vi "Execute.vi"(8 "error in (no error)":errorcluster, 10 "System in":refnum<class "System.lvclass">, 11 "Command in":refnum<class "Command.lvclass">) -> (0 "error out":errorcluster, 3 "Command out":refnum<class "Command.lvclass">)   [LabVIEW 2013, in "Command.lvclass"]
uses:
  Command.lvclass
  Systems/System/System.lvclass
  Command.lvclass/Command.ctl
  States/State/State.lvclass
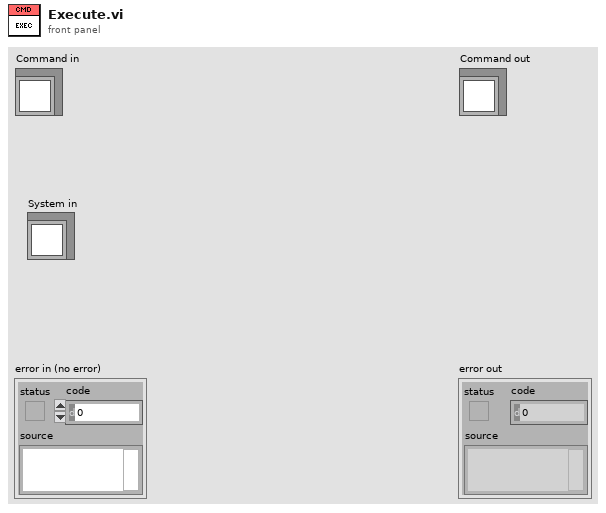
[diagram p1: front panel]
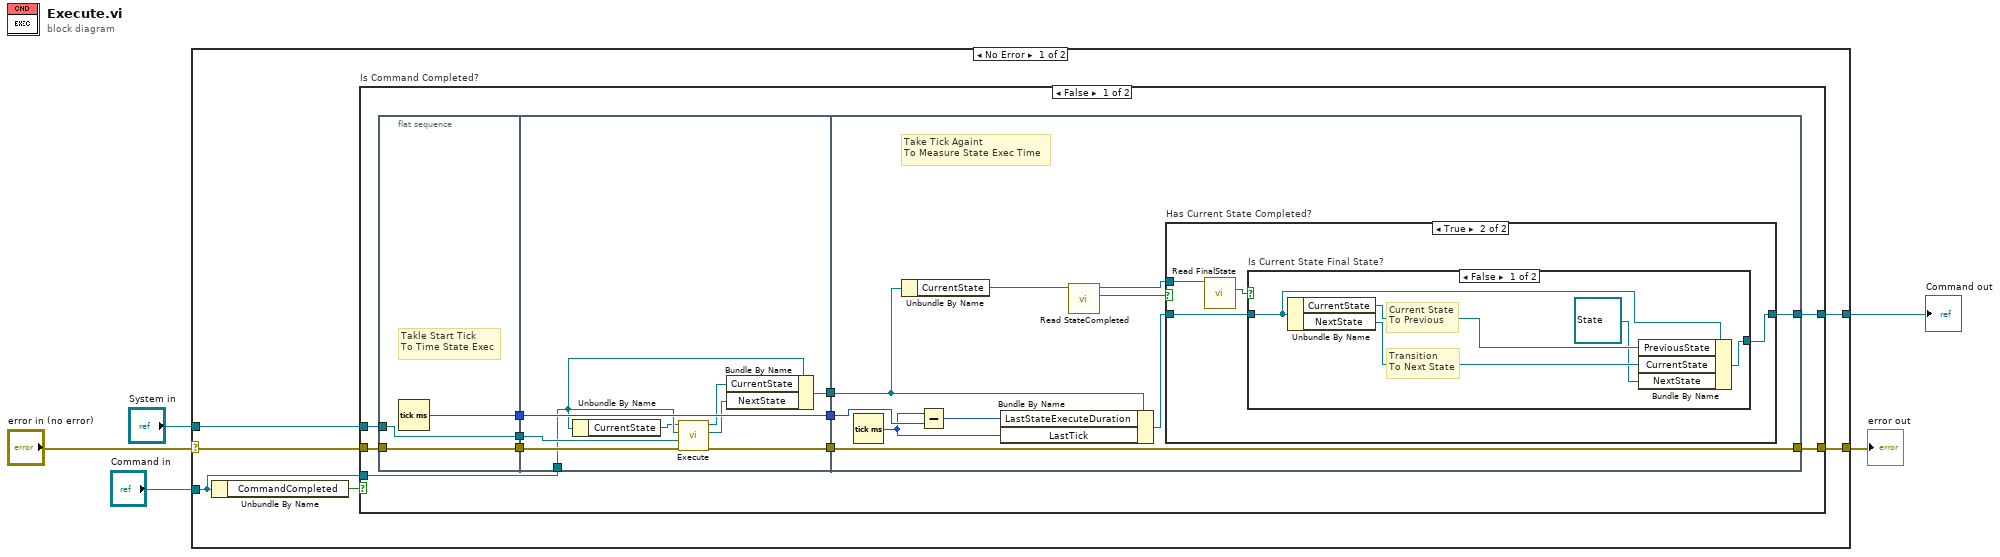
[diagram p0: block diagram]
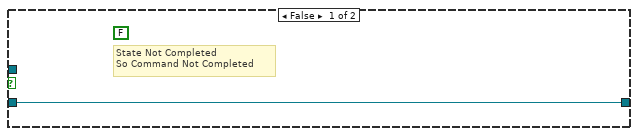
[diagram p2: hidden frame]
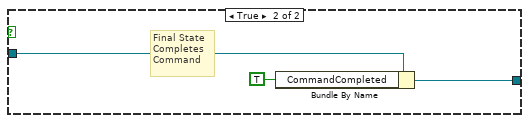
[diagram p3: hidden frame]
diagram:
  n1 = case shown="No Error" "error in (no error)" {
    selector: "error in (no error)" -> [w8 w61]
    tunnel: [w7 w61] -> w4
    tunnel: [w9 w60] -> w2
    tunnel: "Command in" -> [w10 w60]
    tunnel: "System in" -> [w6 _]
    frame No Error {
      n2 = Unbundle By Name(w10) -> ("CommandCompleted"=w11:bool)
      n3 = case "Is Command Completed?" shown="False" w11 {
        tunnel: w10 -> [w13 w58]
        tunnel: [w12 w58] -> w9
        tunnel: w8 -> [w22 w59]
        tunnel: [w21 w59] -> w7
        tunnel: w6 -> [w20 _]
        frame False {
          n4 = flat-sequence {
            tunnel: w20 -> [w24]
            tunnel: w22 -> [w25]
            tunnel: [w25] -> w18
            tunnel: [w24] -> w17
            tunnel: [w23] -> w14
            tunnel: [w33] -> w19
            tunnel: w18 -> [w34]
            tunnel: w17 -> [w32]
            tunnel: [w28] -> w16
            tunnel: [w31] -> w15
            tunnel: w14 -> [w31]
            tunnel: w13 -> [w30]
            tunnel: [w44] -> w21
            tunnel: w19 -> [w44]
            tunnel: w16 -> [w36]
            tunnel: [w38] -> w12
            tunnel: w15 -> [w43]
            frame #0 {
              # "Takle Start Tick\nTo Time State Exec"
              n5 = Tick Count (ms)() -> (millisecond timer value=w23:u32)
            }
            frame #1 {
              n6 = Unbundle By Name(w30) -> ("CurrentState"=w29:refnum<class "State.lvclass">)
              n7 = call-dynamic "Execute.vi"("error in (no error)"=w34, "System in"=w32, "Command in"=w30, "State in"=w29) -> ("error out"=w33:errorcluster, "Next State"=w27:refnum<class "State.lvclass">, "State out"=w26:refnum<class "State.lvclass">)  [unwired: 5 in]
              n8 = Bundle By Name(cluster=w30, "CurrentState"=w26, "NextState"=w27) -> (w28:refnum<class "Command.lvclass">)
            }
            frame #2 {
              # "Take Tick Againt\nTo Measure State Exec Time"
              n9 = Tick Count (ms)() -> (millisecond timer value=w37:u32)
              n10 = Unbundle By Name(w36) -> ("CurrentState"=w35:refnum<class "State.lvclass">)
              n11 = Subtract(x=w37, y=w43) -> (x-y=w42:u32)
              n12 = Bundle By Name(cluster=w36, "LastStateExecuteDuration"=w42, "LastTick"=w37) -> (w39:refnum<class "Command.lvclass">)
              n13 = call-dynamic "Read StateCompleted.vi"("State in"=w35) -> ("StateCompleted"=w41:bool, "State out"=w40:refnum<class "State.lvclass">)  [unwired: 8 in, 1 out]
              n14 = case "Has Current State Completed?" shown="True" w41 {
                tunnel: w39 -> [w45 w47]
                tunnel: w40 -> [_ w49]
                tunnel: [w45 w46] -> w38
                frame False {
                  (unwired) FALSE
                  # "State Not Completed\nSo Command Not Completed"
                }
                frame True {
                  n15 = call-dynamic "Read FinalState.vi"("State in"=w49) -> ("FinalState"=w48:bool)  [unwired: 8 in, 2 out]
                  n16 = case "Is Current State Final State?" shown="False" w48 {
                    tunnel: w47 -> [w53 w57]
                    tunnel: [w54 w56] -> w46
                    frame False {
                      # "Current State\nTo Previous"
                      # "Transition \nTo Next State"
                      n17 = Unbundle By Name(w53) -> ("CurrentState"=w52:refnum<class "State.lvclass">, "NextState"=w51:refnum<class "State.lvclass">)
                      n18 = Bundle By Name(cluster=w53, "PreviousState"=w52, "CurrentState"=w51, "NextState"=refnum<class "State.lvclass"> refnum ("State.lvclass")) -> (w54:refnum<class "Command.lvclass">)
                    }
                    frame True {
                      # "Final State \nCompletes \nCommand"
                      n19 = Bundle By Name(cluster=w57, "CommandCompleted"=TRUE) -> (w56:refnum<class "Command.lvclass">)
                    }
                  }
                }
              }
            }
          }
        }
        frame True {
          # "If Completed, Don't Execute State"
        }
      }
    }
    frame Error {
    }
  }
  "error out" <- w4
  "Command out" <- w2
